vi "Instrumento_caracterizacion_2.vi"() -> ()   [LabVIEW 2009]
uses:
  <vilib>/Analysis/NI_AALBase.lvlib
panel:
  in  "Seleción método":bool
  out "?":bool
  out "?":bool
  out "?":bool
  out "?":bool
  out "?":bool
  out "?":bool
  out "?":bool
  out "?":bool
  out "Secuencia de medidas para caracterización":string[](array[string])=["I1", "I2", "I3", "I'3", "I7", "I'7", "I6", "I5", "I'4", "I4"]
  out "?":bool
  out "?":bool
  in  "Activate switches":bool
  out "Numeric":dbl
  out "Numeric 2":dbl
  in  "Array 3":bool[](array[boolean])
  in  "Amp vs ng":bool
  in  "fas vs ng":bool
  in  "Directorio scripts matlab 2":path=path "C:/Users/franjas/Documents/rutinas-calibracion-slm"
  in  "Exit live":bool
  in  "Capture":bool
  in  "stop":bool
  in  "File to load":path
  in  "File to save":path
  in  "VCD Properties":bool
  in  "Save properties":bool
  in  "Load properties":bool
  in  "Configurar para franjas":bool
  out "Histogram Graph":T1(graph)
  in  "Run live preview":bool
  out "Live Picture":picture
  out "Video formats":string[](array[string])
  out "Devices":string[](array[string])
  in  "ICImagingControl":refnum<k7>(container)
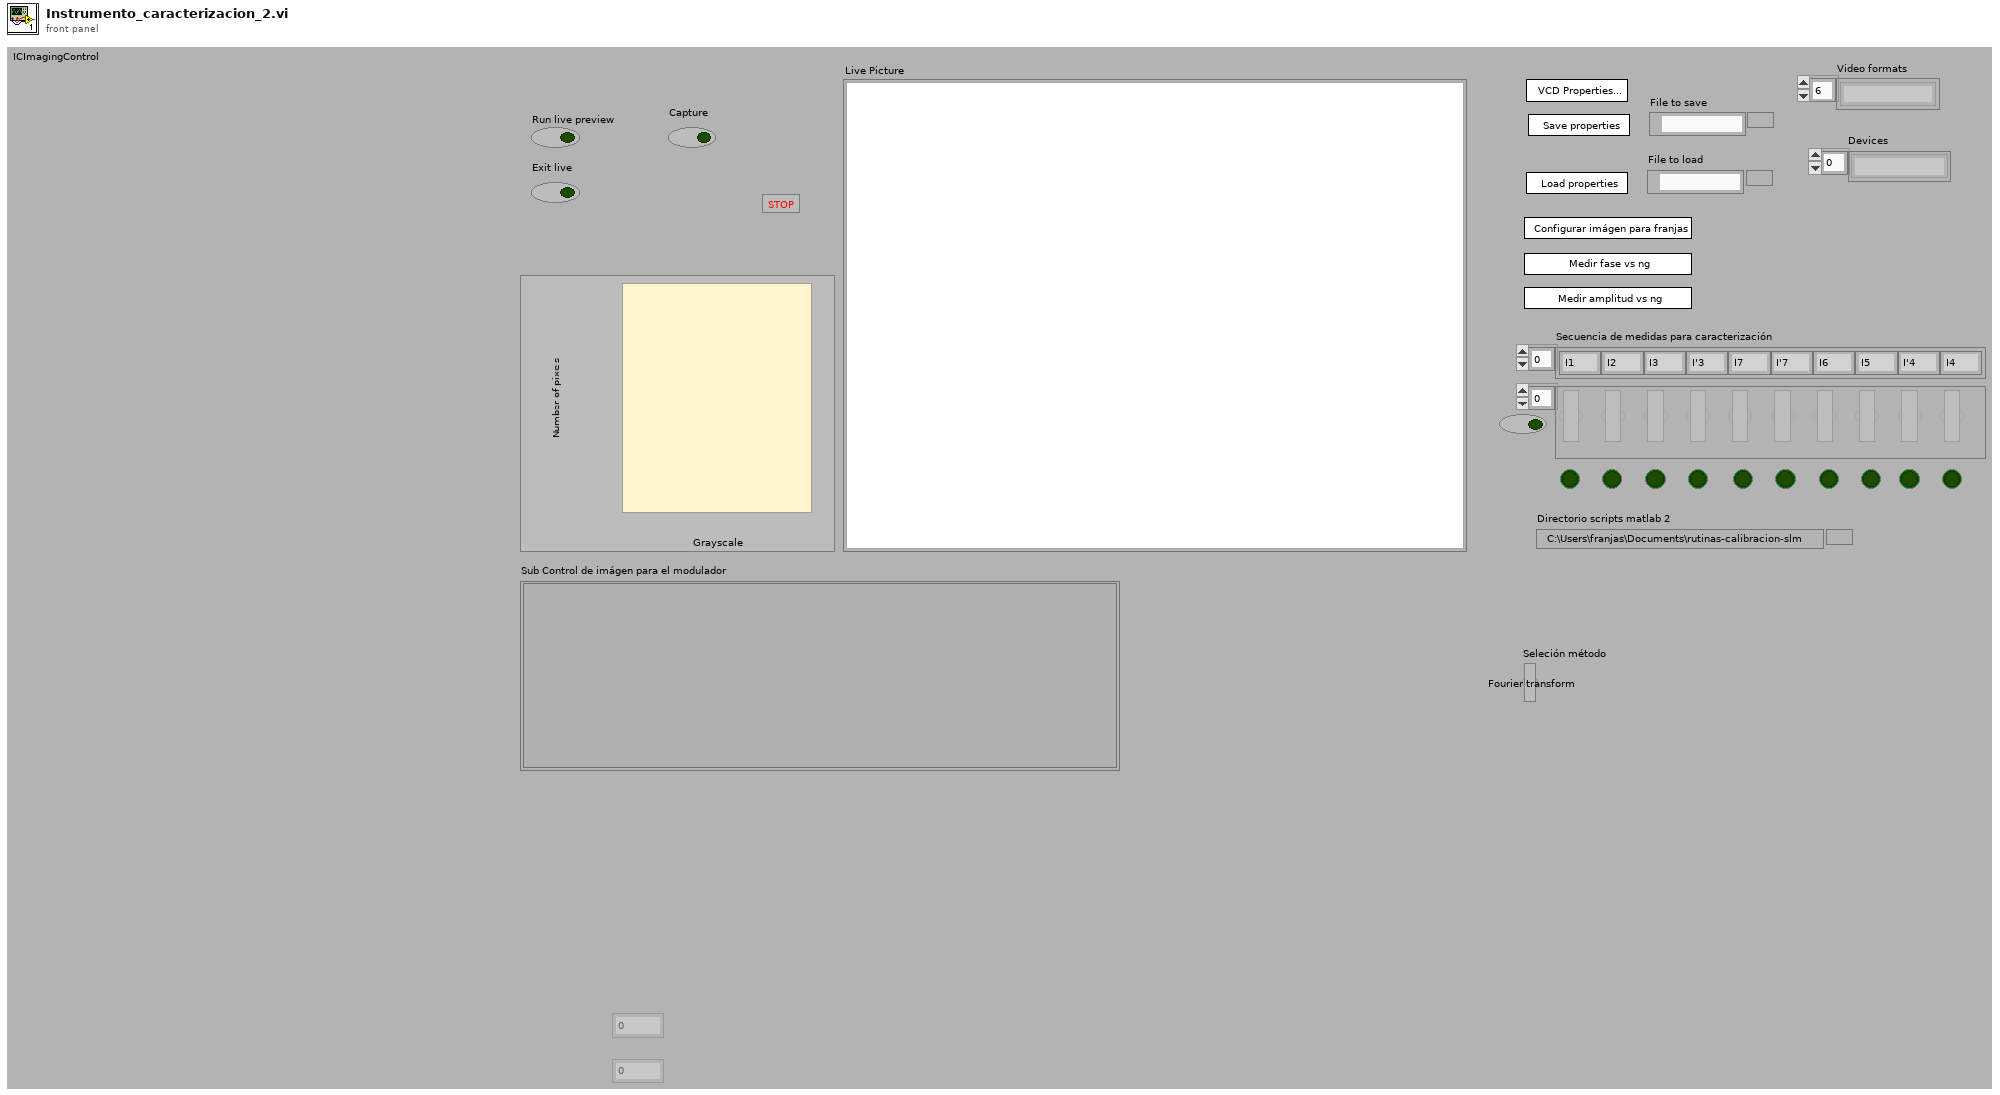
[diagram p1: front panel]
types:
  T1 = cluster{"X Values":dbl[], "Histogram: h(x)":i32[]}
  T2 = typedef "imagedata.ctl" = cluster{"image type":i32, "image depth":i32, "image":u8[], "mask":u8[], "colors":u32[], "Rectangle":cluster{"left":i16, "top":i16, "right":i16, "bottom":i16}}
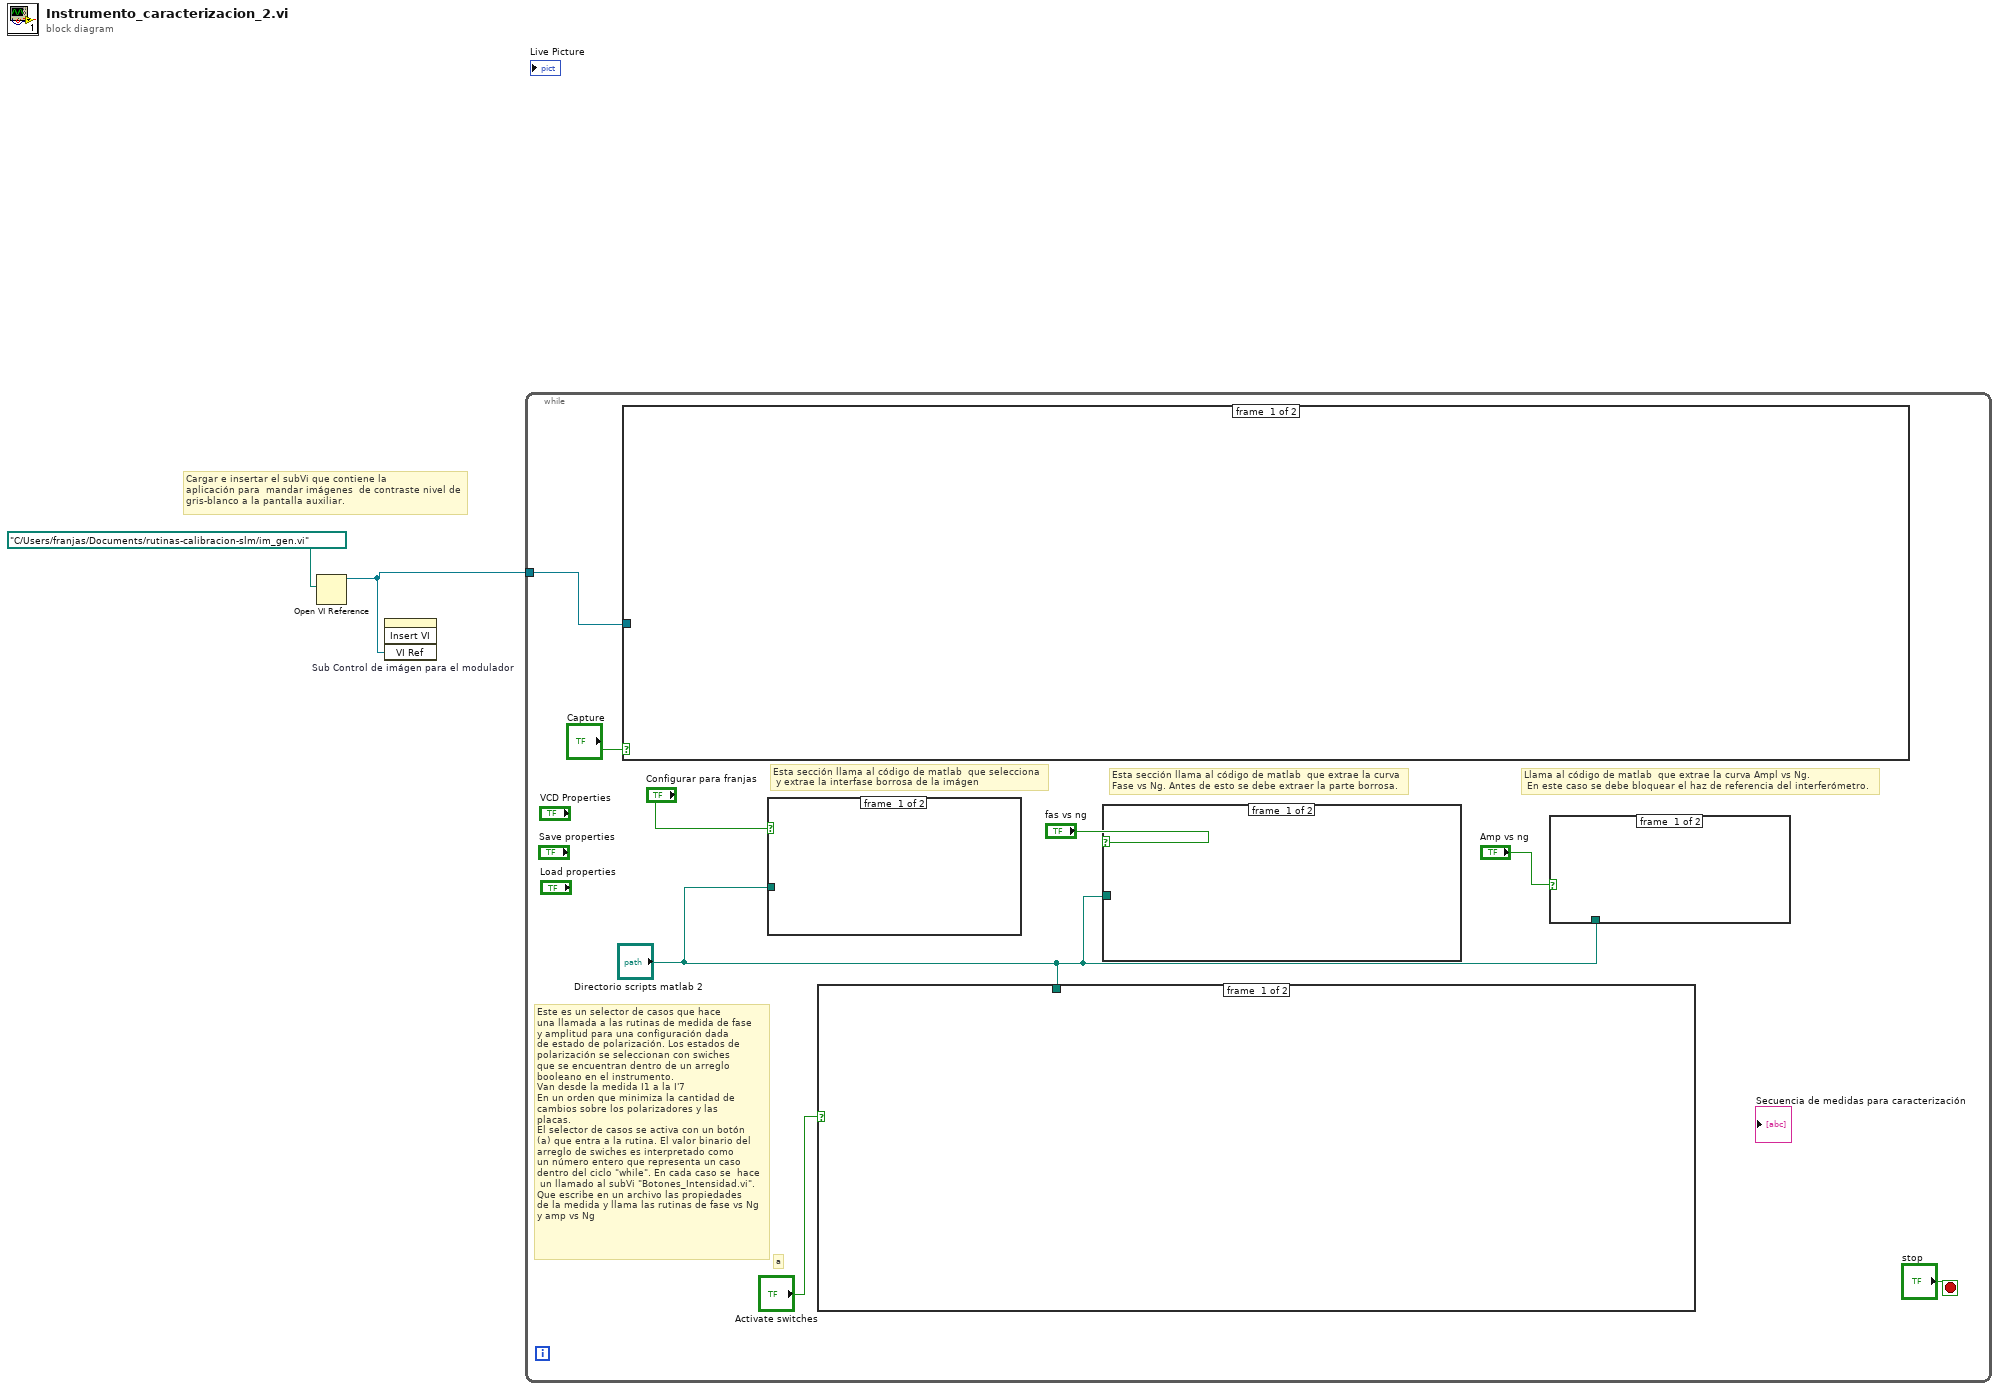
[diagram p0: block diagram]
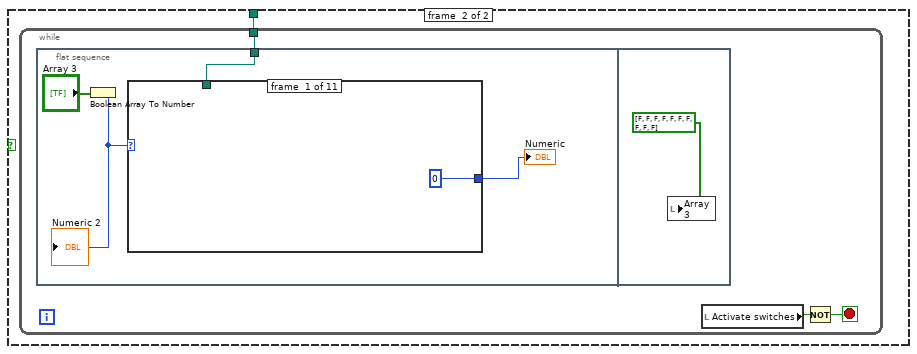
[diagram p2: hidden frame]
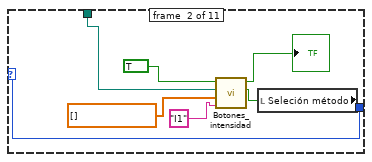
[diagram p3: hidden frame]
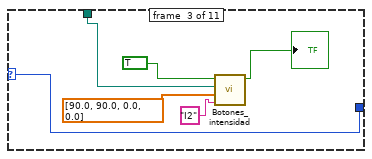
[diagram p4: hidden frame]
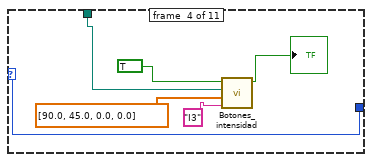
[diagram p5: hidden frame]
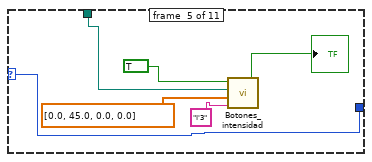
[diagram p6: hidden frame]
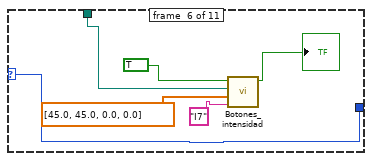
[diagram p7: hidden frame]
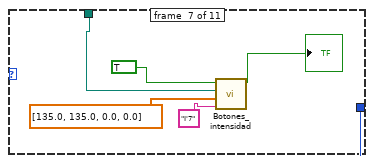
[diagram p8: hidden frame]
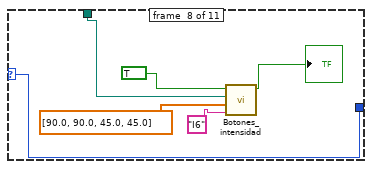
[diagram p9: hidden frame]
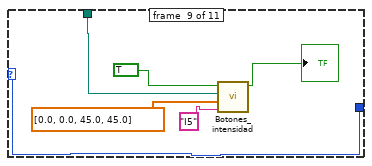
[diagram p10: hidden frame]
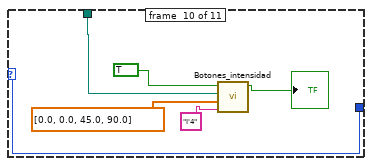
[diagram p11: hidden frame]
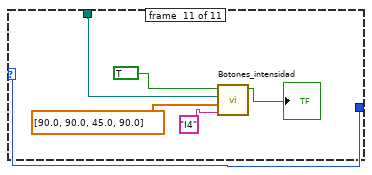
[diagram p12: hidden frame]
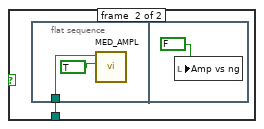
[diagram p13: hidden frame]
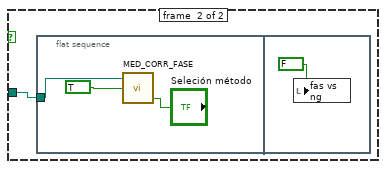
[diagram p14: hidden frame]
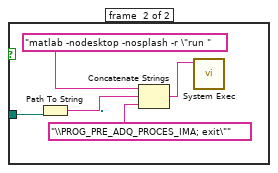
[diagram p15: hidden frame]
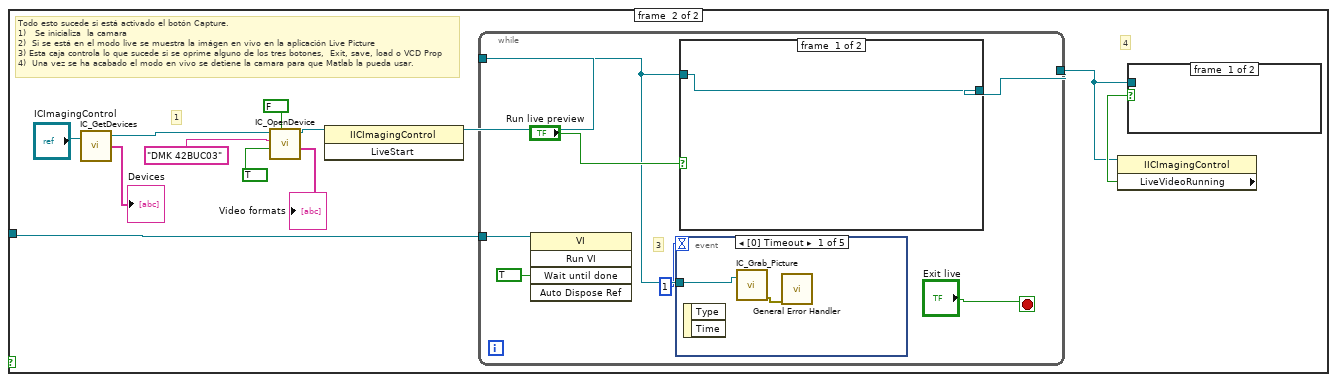
[diagram p16: hidden frame]
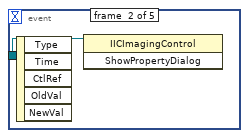
[diagram p17: hidden frame]
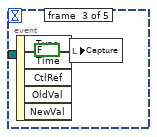
[diagram p18: hidden frame]
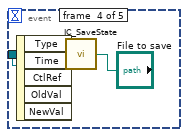
[diagram p19: hidden frame]
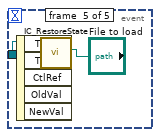
[diagram p20: hidden frame]
diagram:
  # "Cargar e insertar el subVi que contiene la \naplicación para  mandar imágenes  de contraste nivel de gris-blanco a la pantalla auxiliar."
  n1 = Open VI Reference(vi path=path "C:/Users/franjas/Documents/rutinas-calibracion-slm/im_gen.vi") -> (vi reference=w1:refnum<vi>)  [unwired: 5 in, 1 out]
  n2 = invoke on="Sub Control de imágen para el modulador" class="SubPanel" method="Insert VI"("VI Ref"=w1) -> ()  [unwired: 3 in, 4 out]
  n3 = while {
    tunnel: w1 -> [w7]
    stop <- "stop" stop-if-true
    # "a"
    # "Este es un selector de casos que hace\nuna llamada a las rutinas de medida de fase\ny amplitud para una configuración dada \nde estado de polarización. Los estados de\npolarización se seleccionan con swiches\nque se encuentran dentro de un arreglo \nbooleano en el instrumento. \nVan desde la medida I1 a la I'7\nEn un orden que minimiza la cantidad de \ncambios sobre los polarizadores y las \nplacas.\nEl selector de casos se activa con un botón\n(a) que entra a la rutina. El valor binario del \narreglo de swiches es interpretado como\nun número entero que representa un caso \ndentro del ciclo \"while\". En cada caso se  hace\n un llamado al subVi \"Botones_Intensidad.vi\".\nQue escribe en un archivo las propiedades\nde la medida y llama las rutinas de fase vs Ng\ny amp vs Ng"
    # "Llama al código de matlab  que extrae la curva Ampl vs Ng.\n En este caso se debe bloquear el haz de referencia del interferómetro."
    # "Esta sección llama al código de matlab  que extrae la curva\nFase vs Ng. Antes de esto se debe extraer la parte borrosa."
    # "Esta sección llama al código de matlab  que selecciona\n y extrae la interfase borrosa de la imágen"
    n4 = case shown="True" "Capture" {
      tunnel: w7 -> [_ w96]
      frame #0 {
      }
      frame #1 {
        # "4"
        # "1"
        # "Todo esto sucede si está activado el botón Capture.  \n1)   Se inicializa  la camara \n2)  Si se está en el modo live se muestra la imágen en vivo en la aplicación Live Picture\n3) Esta caja controla lo que sucede si se oprime alguno de los tres botones,  Exit, save, load o VCD Prop\n4)  Una vez se ha acabado el modo en vivo se detiene la camara para que Matlab la pueda usar."
        n5 = call <userlib>:"IC_GetDevices.vi"("ICImagingControl In"="ICImagingControl") -> ("ICImagingControl Out"=w105:refnum<k7>, "Devices"=→"Devices":string[])  [unwired: 1 in, 1 out]
        n6 = call <userlib>:"IC_OpenDevice.vi"("Color"=FALSE, "Live"=TRUE, "Device"="DMK 42BUC03", "ICImagingControl In"=w105) -> ("VideoFormats"=→"Video formats":string[], "ICImagingControl Out"=w99:refnum<k7>)  [unwired: 2 in, 4 out]
        n7 = invoke class="IICImagingControl" method="LiveStart"(reference=w99) -> (reference out=w97:refnum<k7>)  [unwired: 2 in, 2 out]
        n8 = while {
          tunnel: w97 -> [w109]
          tunnel: [w114] -> w98
          tunnel: w96 -> [w111]
          stop <- "Exit live" stop-if-true
          # "3"
          n9 = invoke class="VI" method="Run VI"(reference=w111, "Wait until done"=TRUE ("Wait Until Done")) -> ()  [unwired: 3 in, 5 out]
          n10 = event shown="[0] Timeout" {
            selector: _ -> [_ _ _ _ _]
            dyn-events: _ -> [_ _ _ _ _]
            timeout: 1 -> [_ _ _ _ _]
            tunnel: w109 -> [w115 w117 _ w120 w122]
            event #0 {
              n11 = event-data() -> ()  [unwired: 1 in, 2 out]
              n12 = call <userlib>:"IC_Grab_Picture.vi"("ICImagingControl In"=w115) -> ("Error Out"=w116:errorcluster)  [unwired: 1 in, 3 out]
              n13 = call <vilib>:"General Error Handler.vi"("error in (no error)"=w116) -> ()  [unwired: 10 in, 5 out]
            }
            event #1 {
              n14 = event-data() -> ()  [unwired: 1 in, 5 out]
              n15 = invoke class="IICImagingControl" method="ShowPropertyDialog"(reference=w117) -> ()  [unwired: 2 in, 3 out]
            }
            event #2 {
              n16 = event-data() -> ()  [unwired: 1 in, 5 out]
              n17 = local write "Capture"(FALSE ("CApture")) -> ()
            }
            event #3 {
              n18 = event-data() -> ()  [unwired: 1 in, 5 out]
              n19 = call <userlib>:"IC_SaveState.vi"("file path"="File to save", "ICImagingControl In"=w120) -> ()  [unwired: 1 in, 2 out]
            }
            event #4 {
              n20 = event-data() -> ()  [unwired: 1 in, 5 out]
              n21 = call <userlib>:"IC_RestoreState.vi"("File Path"="File to load", "ICImagingControl"=w122) -> ()  [unwired: 2 in, 2 out]
            }
          }
          n22 = case shown="True" "Run live preview" {
            tunnel: w109 -> [w123 w129]
            tunnel: [w123 w124] -> w114
            frame #0 {
            }
            frame #1 {
              # "2"
              n23 = call <userlib>:"IC_Grab_Picture.vi"("ICImagingControl In"=w129) -> ("ICImagingControl Out"=w124:refnum<k7>, "Picture Out"=w132:picture)  [unwired: 1 in, 2 out]
              n24 = call <vilib>:"Picture to Pixmap.vi"("depth"=24, "picture"=w132) -> ("image data"=w128:T2)  [unwired: 8 in, 1 out]
              n25 = Unbundle By Name(w128) -> ("image"=w127:u8[])
              n26 = call <vilib>:"Draw Flattened Pixmap.vi"("image data"=w128) -> ("new picture"=w130:picture)  [unwired: 8 in]
              n27 = local write "Live Picture"(w130) -> ()
              n28 = call <vilib>:"Histogram.vi"("intervals"=100, "X"=w127) -> ("Histogram Graph"=→"Histogram Graph":T1)  [unwired: 6 in, 3 out]
            }
          }
        }
        n29 = property class="IICImagingControl"(reference=w98) -> ("LiveVideoRunning"=w100:bool)  [unwired: 1 in, 2 out]
        n30 = case shown="True" w100 {
          tunnel: w98 -> [_ w133]
          frame #0 {
          }
          frame #1 {
            n31 = invoke class="IICImagingControl" method="LiveStop"(reference=w133) -> ()  [unwired: 2 in, 3 out]
          }
        }
      }
    }
    n32 = case shown="False" "Configurar para franjas" {
      tunnel: "Directorio scripts matlab 2" -> [_ w91]
      frame #0 {
      }
      frame #1 {
        n33 = Path To String(path=w91) -> (string=w95:string)
        n34 = Concatenate Strings("matlab -nodesktop -nosplash -r \"run " ("command line"), w95, "\\PROG_PRE_ADQ_PROCES_IMA; exit\"" ("command line")) -> (w94:string)
        n35 = call <vilib>:"System Exec.vi"("command line"=w94) -> ()  [unwired: 7 in, 4 out]
      }
    }
    n36 = case shown="True" "Activate switches" {
      tunnel: "Directorio scripts matlab 2" -> [_ w11]
      frame #0 {
      }
      frame #1 {
        n37 = while {
          tunnel: w11 -> [w12]
          stop <- w14 stop-if-true
          n38 = flat-sequence {
            tunnel: w12 -> [w15]
            frame #0 {
              n39 = Boolean Array To Number(Boolean array="Array 3") -> (number=w16:u32)
              "Numeric 2" <- w16
              n40 = case shown="1" w16 {
                selector: w16 -> [_ w26 w32 w38 w44 w50 w56 w62 w68 w74 w80]
                tunnel: [u32 0 w26 w32 w38 w44 w50 w56 w62 w68 w74 w80] -> w18
                tunnel: w15 -> [_ w22 w27 w34 w40 w46 w52 w58 w64 w70 w76]
                frame #0 {
                }
                frame #1 {
                  n41 = local read "Seleción método"() -> (w20:bool)
                  n42 = call "Botones_intensidad.vi"("Seleción método"=w20, "String"="I1", "Array"=dbl[] [] ("Array 4"), "Directorio scripts matlab 2"=w22, "I1"=TRUE) -> (3:→"?":bool)  [unwired: 6 in]
                }
                frame #2 {
                  n43 = call "Botones_intensidad.vi"("String"="I2", "Array"=dbl[] [90.0, 90.0, 0.0, 0.0] ("Array 4"), "Directorio scripts matlab 2"=w27, "I1"=TRUE) -> (3:→"?":bool)  [unwired: 7 in]
                }
                frame #3 {
                  n44 = call "Botones_intensidad.vi"("String"="I3", "Array"=dbl[] [90.0, 45.0, 0.0, 0.0] ("Array 4"), "Directorio scripts matlab 2"=w34, "I1"=TRUE) -> (3:→"?":bool)  [unwired: 7 in]
                }
                frame #4 {
                  n45 = call "Botones_intensidad.vi"("String"="I'3", "Array"=dbl[] [0.0, 45.0, 0.0, 0.0] ("Array 4"), "Directorio scripts matlab 2"=w40, "I1"=TRUE) -> (3:→"?":bool)  [unwired: 7 in]
                }
                frame #5 {
                  n46 = call "Botones_intensidad.vi"("String"="I7", "Array"=dbl[] [45.0, 45.0, 0.0, 0.0] ("Array 4"), "Directorio scripts matlab 2"=w46, "I1"=TRUE) -> (3:→"?":bool)  [unwired: 7 in]
                }
                frame #6 {
                  n47 = call "Botones_intensidad.vi"("String"="I'7", "Array"=dbl[] [135.0, 135.0, 0.0, 0.0] ("Array 4"), "Directorio scripts matlab 2"=w52, "I1"=TRUE) -> (3:→"?":bool)  [unwired: 7 in]
                }
                frame #7 {
                  n48 = call "Botones_intensidad.vi"("String"="I6", "Array"=dbl[] [90.0, 90.0, 45.0, 45.0] ("Array 4"), "Directorio scripts matlab 2"=w58, "I1"=TRUE) -> (3:→"?":bool)  [unwired: 7 in]
                }
                frame #8 {
                  n49 = call "Botones_intensidad.vi"("String"="I5", "Array"=dbl[] [0.0, 0.0, 45.0, 45.0] ("Array 4"), "Directorio scripts matlab 2"=w64, "I1"=TRUE) -> (3:→"?":bool)  [unwired: 7 in]
                }
                frame #9 {
                  n50 = call "Botones_intensidad.vi"("String"="I'4", "Array"=dbl[] [0.0, 0.0, 45.0, 90.0] ("Array 4"), "Directorio scripts matlab 2"=w70, "I1"=TRUE) -> (3:→"?":bool)  [unwired: 7 in]
                }
                frame #10 {
                  n51 = call "Botones_intensidad.vi"("String"="I4", "Array"=dbl[] [90.0, 90.0, 45.0, 90.0] ("Array 4"), "Directorio scripts matlab 2"=w76, "I1"=TRUE) -> (3:→"?":bool)  [unwired: 7 in]
                }
              }
              "Numeric" <- w18
            }
            frame #1 {
              n52 = local write "Array 3"(bool[] [FALSE, FALSE, FALSE, FALSE, FALSE, FALSE, FALSE, FALSE, FALSE, FALSE] ("Array 4")) -> ()
            }
          }
          n53 = local read "Activate switches"() -> (w13:bool)
          n54 = Not(x=w13) -> (.not. x?=w14:bool)
        }
      }
    }
    n55 = case shown="True" "fas vs ng" {
      tunnel: "Directorio scripts matlab 2" -> [_ w86]
      frame #0 {
      }
      frame #1 {
        n56 = flat-sequence {
          tunnel: w86 -> [w89]
          frame #0 {
            n57 = call "MED_CORR_FASE.vi"("Seleción método"="Seleción método", "Ejecucion"=TRUE ("Boolean"), "Directorio scripts matlab"=w89) -> ()
          }
          frame #1 {
            n58 = local write "fas vs ng"(FALSE ("fas vs ng")) -> ()
          }
        }
      }
    }
    n59 = case shown="True" "Amp vs ng" {
      tunnel: "Directorio scripts matlab 2" -> [_ w82]
      frame #0 {
      }
      frame #1 {
        n60 = flat-sequence {
          tunnel: w82 -> [w84]
          frame #0 {
            n61 = call "MED_AMPL.vi"("Boolean"=TRUE, "Directorio scripts matlab"=w84) -> ()  [unwired: 10 in]
          }
          frame #1 {
            n62 = local write "Amp vs ng"(FALSE ("Amp vs ng")) -> ()
          }
        }
      }
    }
  }
